vi "SMTP Email Send Multiple Attachments Charset.vi"(0 "recipients":string[](array[string]), 1 "mail server":string, 2 "return address":string, 3 "character set (us-ascii)":string="us-ascii", 5 "subject ([No Subject])":string="[No Subject]", 7 "message":string, 9 "attachments":T1(array[cluster]), 11 "error in (no error)":errorcluster, 14 "translit":string="MacRoman iso-8859-1 macroman.trl, ToUpper iso-8859-1 toupper.trl,\nMacRomanUp MacRoman toupper.trl") -> (4 "invalid recipients":string[](array[string]), 15 "error out":errorcluster)   [LabVIEW 2009, in "NewNI_SMTPEmail.lvlib"]
doc: "Sends an email with multiple file and data attachments to a list of recipients."
uses:
  NewNI_SMTPEmail.lvlib
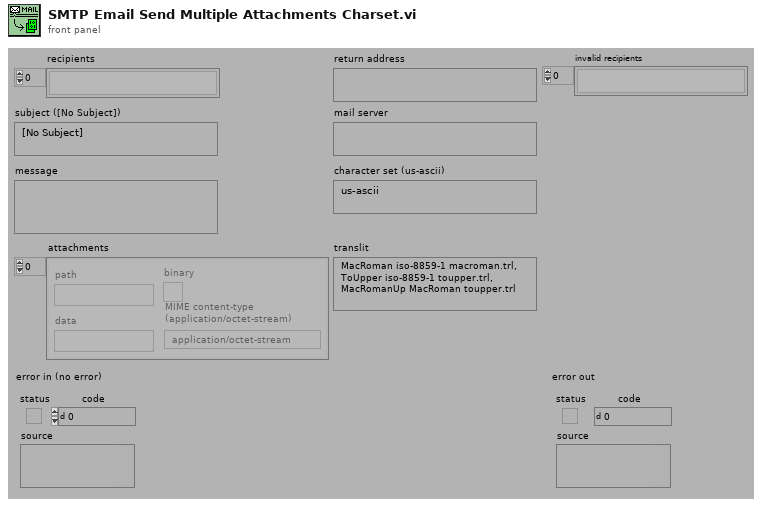
[diagram p1: front panel]
types:
  T1 = cluster{"path":path, "data":string, "binary":bool, "MIME content-type \n(application/octet-stream)":string}[]
  T2 = typedef "NewNI_SMTPEmail.lvlib/SMTP Email Session.ctl" = refnum<k1>
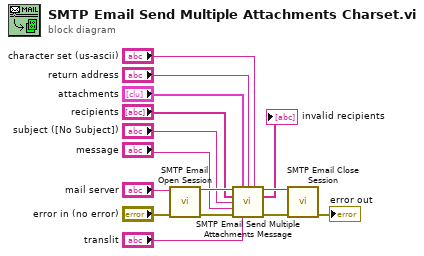
[diagram p0: block diagram]
diagram:
  n1 = call "SMTP Email Open Session.vi"("error in (no error)"="error in (no error)", "mail server"="mail server") -> ("error out"=w14:errorcluster, "smtp session out"=w13:T2)  [unwired: 1 in, 3 out]
  n2 = call "SMTP Email Send Multiple Attachments Message.vi"("smtp session"=w13, "attachments"="attachments", "return address"="return address", "character set"="character set (us-ascii)", "recipients"="recipients", "subject"="subject ([No Subject])", "message"="message", "error in (no error)"=w14, "translit"="translit") -> ("smtp session out"=w12:T2, "invalid recipients"=→"invalid recipients":string[], "error out"=w11:errorcluster)  [unwired: 4 out]
  n3 = call "SMTP Email Close Session.vi"("error in (no error)"=w11, "smtp session"=w12) -> ("error out"=→"error out":errorcluster)  [unwired: 5 out]
